vi "Dresser DXD Temp and Press Read Standalone.vi"(0 "Serial Port (COM1)":refnum<visa-resource-name>="COM1", 1 "Serial Baud Rate (19200)":u16(ring)=4 items=["1200", "2400", "4800", "9600", "19200", "38400", "57600", "115200"], 5 "DXD Address (1)":T2=1 min=1 max=99 step=1, 7 "Pressure Units (PSI)":T1(ring), 11 "Error In (no error)":errorcluster) -> (6 "Current Pressure":dbl min=-999999.0 max=999999.0 step=1e-05 format="%.2f", 8 "Current Temperature":dbl caption="°C" min=-999999.0 max=999999.0 step=1e-05 format="%.3f", 10 "Pressure Type":string, 15 "Error Out":errorcluster)   [LabVIEW 2015]
doc: "This getting started VI demonstrates how to continuously retrieve a pressure reading, with the selected units, and a temperature reading from the Dresser DXD Series pressure transducer at the specified address.\n\nSelect the serial port, serial baud rate, and DXD address prior to clicking the run arrow. \nThe pressure units selection can be changed while running.\nWritten by:\nBLOOMY CONTROLS, INC\nWINDSOR, CT 06095, USA\n860-298-9925\nwww.bloomy.com\nV2.0.0\nMay, 2002"
uses:
  Type Defs/DXD Address.ctl
panel:
  out "Heise Label (S/N)":string="000000"
  in  "Termination Character (T, <lf>)":bool=TRUE caption="<lf>\n<cr>"
  in  "Serial Stop Bits (1)":u16(ring)=10 items=["1.0"=10, "1.5"=15, "2.0"=20]
  in  "Serial Parity (even)":u16(ring)=2 items=["None", "Odd", "Even", "Mark", "Space"]
  in  "Serial Flow Control (None)":u16(ring) items=["None"=0, "XON/XOFF"=1, "RTS/CTS"=2, "DTR/DSR"=4]
  in  "Serial Data Bits (7)":u16=7
  out "Pressure Units":T1(ring)
  # "For instructions on the use of this VI, press Ctrl+H to display the help window and move the mouse over the icon, controls, and indicators"
  # "<---the unit selection can be changed while running"
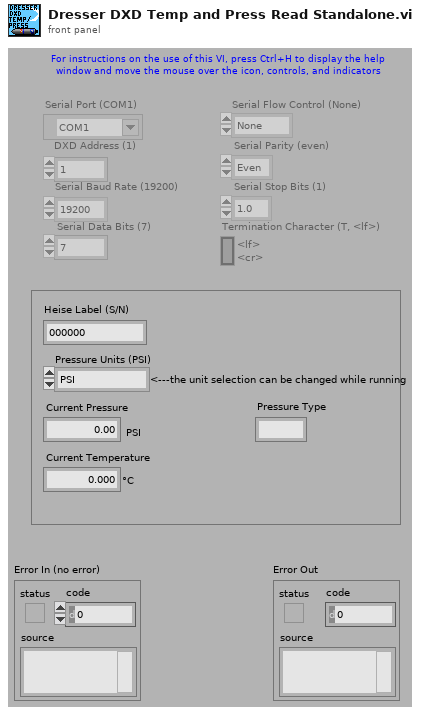
[diagram p1: front panel]
types:
  T1 = enum16{"PSI", "Bar", "cm H2O", "ft H2O", "hectoPascal", "in Hg", "in H2O", "kiloPascal", "milliBar", "mmHg", "MegaPascal", "Numeric Pressure"}
  T2 = typedef "DXD Address.ctl" = i32
  T3 = enum16{"Error status character set in bit 1 is returned", "No error status character (legacy mode)"}
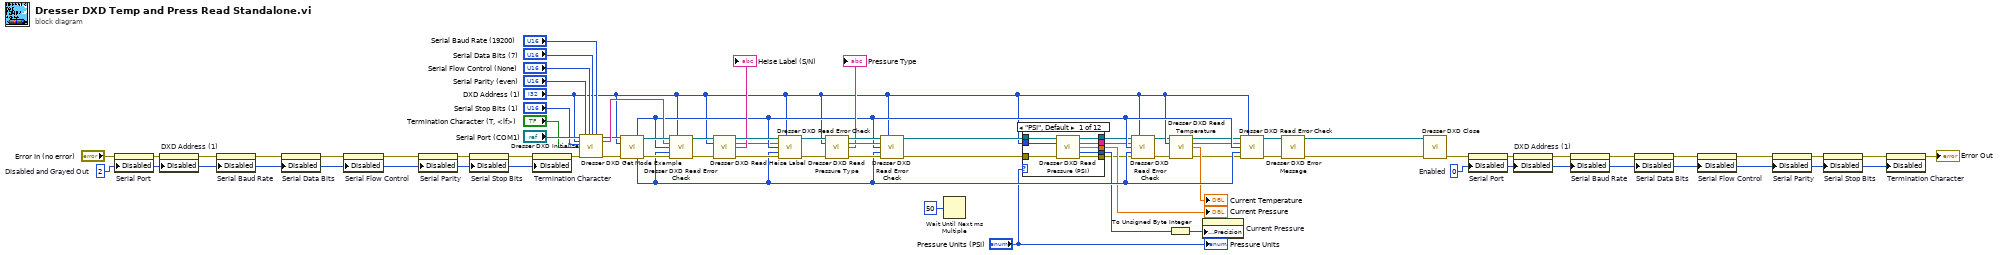
[diagram p0: block diagram]
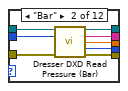
[diagram p2: hidden frame]
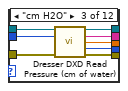
[diagram p3: hidden frame]
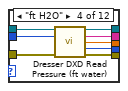
[diagram p4: hidden frame]
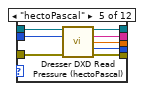
[diagram p5: hidden frame]
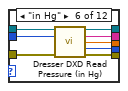
[diagram p6: hidden frame]
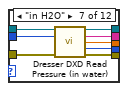
[diagram p7: hidden frame]
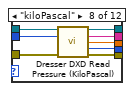
[diagram p8: hidden frame]
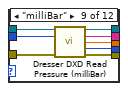
[diagram p9: hidden frame]
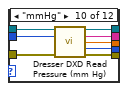
[diagram p10: hidden frame]
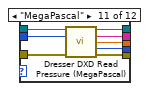
[diagram p11: hidden frame]
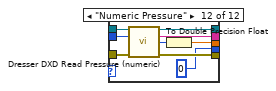
[diagram p12: hidden frame]
diagram:
  w39 = u8 0  # Enabled
  w45 = u8 2  # Disabled and Grayed Out
  n1 = property on="Serial Port" class="VISAName"(error in="Error In (no error)", "Disabled"=w45) -> (error out=w48:errorcluster)  [unwired: 1 in, 1 out]
  n2 = property on="DXD Address (1)" class="DigNum (strict)"(error in=w48, "Disabled"=w45) -> (error out=w47:errorcluster)  [unwired: 1 in, 1 out]
  n3 = property on="Serial Baud Rate" class="Ring (strict)"(error in=w47, "Disabled"=w45) -> (error out=w46:errorcluster)  [unwired: 1 in, 1 out]
  n4 = property on="Serial Data Bits" class="DigNum (strict)"(error in=w46, "Disabled"=w45) -> (error out=w44:errorcluster)  [unwired: 1 in, 1 out]
  n5 = property on="Serial Flow Control" class="Ring (strict)"(error in=w44, "Disabled"=w45) -> (error out=w43:errorcluster)  [unwired: 1 in, 1 out]
  n6 = property on="Serial Parity" class="Ring (strict)"(error in=w43, "Disabled"=w45) -> (error out=w42:errorcluster)  [unwired: 1 in, 1 out]
  n7 = property on="Serial Stop Bits" class="Ring (strict)"(error in=w42, "Disabled"=w45) -> (error out=w41:errorcluster)  [unwired: 1 in, 1 out]
  n8 = property on="Termination Character" class="Bool (strict)"(error in=w41, "Disabled"=w45) -> (error out=w40:errorcluster)  [unwired: 1 in, 1 out]
  n9 = call "Dresser DXD Initialize.vi"("Serial Port (COM1)"="Serial Port (COM1)", "DXD Address (1)"="DXD Address (1)", "Serial Stop Bits (1)"="Serial Stop Bits (1)", "Termination Character (T, <lf>)"="Termination Character (T, <lf>)", "error in (no error)"=w40, "Serial Parity (even)"="Serial Parity (even)", "Serial Flow Control (None)"="Serial Flow Control (None)", "Serial Data Bits (7)"="Serial Data Bits (7)", "Serial Baud Rate (19200)"="Serial Baud Rate (19200)") -> ("VISA session"=w28:refnum<visa-resource-name>, "Returned String"=w61:string, "Error Out"=w29:errorcluster)  [unwired: 8 in]
  n10 = call "Dresser DXD Get Mode Example.vi"("VISA session"=w28, "DXD Address (1)"="DXD Address (1)", "Error In (no error)"=w29) -> ("Bit 1 - Error Status Character"=w19:enum16{"ACK/NAK", "A/N"}, "dup VISA session"=w63:refnum<visa-resource-name>, "Bit 5 - Error Status Character"=w20:T3, "Error Out"=w62:errorcluster)  [unwired: 2 in, 7 out]
  n11 = call "Dresser DXD Read Error Check.vi"("VISA session"=w63, "DXD Address (1)"="DXD Address (1)", "Returned String (\"\")"=w61, "Mode Bit 1 - Error Status Character"=w19, "Mode Bit 5 - Error Status Character"=w20, "Error In (no error)"=w62) -> ("dup VISA session"=w27:refnum<visa-resource-name>, "Error Out"=w26:errorcluster)  [unwired: 6 in, 2 out]
  n12 = call "Dresser DXD Read Heise Label.vi"("VISA session"=w27, "DXD Address (1)"="DXD Address (1)", "Error In (no error)"=w26) -> ("dup VISA session"=w25:refnum<visa-resource-name>, "Returned String"=w18:string, "Heise Label (S/N)"=→"Heise Label (S/N)":string, "Error Out"=w24:errorcluster)  [unwired: 9 in]
  n13 = call "Dresser DXD Read Error Check.vi"("VISA session"=w25, "DXD Address (1)"="DXD Address (1)", "Returned String (\"\")"=w18, "Mode Bit 1 - Error Status Character"=w19, "Mode Bit 5 - Error Status Character"=w20, "Error In (no error)"=w24) -> ("dup VISA session"=w23:refnum<visa-resource-name>, "Error Out"=w22:errorcluster)  [unwired: 6 in, 2 out]
  n14 = call "Dresser DXD Read Pressure Type.vi"("VISA session"=w23, "DXD Address (1)"="DXD Address (1)", "Error In (no error)"=w22) -> ("dup VISA session"=w58:refnum<visa-resource-name>, "Returned String"=w56:string, "Pressure Type"=→"Pressure Type":string, "Error Out"=w60:errorcluster)  [unwired: 9 in]
  n15 = call "Dresser DXD Read Error Check.vi"("VISA session"=w58, "DXD Address (1)"="DXD Address (1)", "Returned String (\"\")"=w56, "Mode Bit 1 - Error Status Character"=w19, "Mode Bit 5 - Error Status Character"=w20, "Error In (no error)"=w60) -> ("dup VISA session"=w57:refnum<visa-resource-name>, "Error Out"=w59:errorcluster)  [unwired: 6 in, 2 out]
  n16 = Wait Until Next ms Multiple(millisecond multiple=u32 50) -> ()  [unwired: 1 out]
  n17 = case shown="\"PSI\", Default" "Pressure Units (PSI)" {
    tunnel: [w75 w78 w86 w94 w102 w110 w118 w126 w134 w142 w150 w160] -> w5
    tunnel: [w74 w81 w89 w97 w105 w113 w121 w129 w137 w145 w153 w162] -> w4
    tunnel: w57 -> [w73 w83 w91 w99 w107 w115 w123 w131 w139 w147 w155 w164]
    tunnel: w59 -> [w72 w82 w90 w98 w106 w114 w122 w130 w138 w146 w154 w163]
    tunnel: "DXD Address (1)" -> [w71 w77 w85 w93 w101 w109 w117 w125 w133 w141 w149 w159]
    tunnel: [w70 w80 w88 w96 w104 w112 w120 w128 w136 w144 w152 0 ("Pressure Decimal Position")] -> w14
    tunnel: [w69 w79 w87 w95 w103 w111 w119 w127 w135 w143 w151 w156] -> w13
    tunnel: [w68 w76 w84 w92 w100 w108 w116 w124 w132 w140 w148 w157] -> w1
    frame "PSI", Default {
      n18 = call "Dresser DXD Read Pressure (PSI).vi"("VISA session"=w73, "DXD Address (1)"=w71, "Error In (no error)"=w72) -> ("dup VISA session"=w75:refnum<visa-resource-name>, "Returned String"=w68:string, "Current Pressure (PSI)"=w69:dbl, "Pressure Decimal Position"=w70:i32, "Error Out"=w74:errorcluster)  [unwired: 8 in]
    }
    frame "Bar" {
      n19 = call "Dresser DXD Read Pressure (Bar).vi"("VISA session"=w83, "DXD Address (1)"=w77, "Error In (no error)"=w82) -> ("dup VISA session"=w78:refnum<visa-resource-name>, "Returned String"=w76:string, "Current Pressure (Bar)"=w79:dbl, "Pressure Decimal Position"=w80:i32, "Error Out"=w81:errorcluster)  [unwired: 8 in]
    }
    frame "cm H2O" {
      n20 = call "Dresser DXD Read Pressure (cm of water).vi"("VISA session"=w91, "DXD Address (1)"=w85, "Error In (no error)"=w90) -> ("dup VISA session"=w86:refnum<visa-resource-name>, "Returned String"=w84:string, "Current Pressure (cm of water)"=w87:dbl, "Pressure Decimal Position"=w88:i32, "Error Out"=w89:errorcluster)  [unwired: 8 in]
    }
    frame "ft H2O" {
      n21 = call "Dresser DXD Read Pressure (ft water).vi"("VISA session"=w99, "DXD Address (1)"=w93, "Error In (no error)"=w98) -> ("dup VISA session"=w94:refnum<visa-resource-name>, "Returned String"=w92:string, "Current Pressure (ft water)"=w95:dbl, "Pressure Decimal Position"=w96:i32, "Error Out"=w97:errorcluster)  [unwired: 8 in]
    }
    frame "hectoPascal" {
      n22 = call "Dresser DXD Read Pressure (hectoPascal).vi"("VISA session"=w107, "DXD Address (1)"=w101, "Error In (no error)"=w106) -> ("dup VISA session"=w102:refnum<visa-resource-name>, "Returned String"=w100:string, "Current Pressure (hectoPascal)"=w103:dbl, "Pressure Decimal Position"=w104:i32, "Error Out"=w105:errorcluster)  [unwired: 8 in]
    }
    frame "in Hg" {
      n23 = call "Dresser DXD Read Pressure (in Hg).vi"("VISA session"=w115, "DXD Address (1)"=w109, "Error In (no error)"=w114) -> ("dup VISA session"=w110:refnum<visa-resource-name>, "Returned String"=w108:string, "Current Pressure (in Hg)"=w111:dbl, "Pressure Decimal Position"=w112:i32, "Error Out"=w113:errorcluster)  [unwired: 8 in]
    }
    frame "in H2O" {
      n24 = call "Dresser DXD Read Pressure (in water).vi"("VISA session"=w123, "DXD Address (1)"=w117, "Error In (no error)"=w122) -> ("dup VISA session"=w118:refnum<visa-resource-name>, "Returned String"=w116:string, "Current Pressure (in H2O)"=w119:dbl, "Pressure Decimal Position"=w120:i32, "Error Out"=w121:errorcluster)  [unwired: 8 in]
    }
    frame "kiloPascal" {
      n25 = call "Dresser DXD Read Pressure (KiloPascal).vi"("VISA session"=w131, "DXD Address (1)"=w125, "Error In (no error)"=w130) -> ("dup VISA session"=w126:refnum<visa-resource-name>, "Returned String"=w124:string, "Current Pressure (KiloPascal)"=w127:dbl, "Pressure Decimal Position"=w128:i32, "Error Out"=w129:errorcluster)  [unwired: 8 in]
    }
    frame "milliBar" {
      n26 = call "Dresser DXD Read Pressure (milliBar).vi"("VISA session"=w139, "DXD Address (1)"=w133, "Error In (no error)"=w138) -> ("dup VISA session"=w134:refnum<visa-resource-name>, "Returned String"=w132:string, "Current Pressure (milliBar)"=w135:dbl, "Pressure Decimal Position"=w136:i32, "Error Out"=w137:errorcluster)  [unwired: 8 in]
    }
    frame "mmHg" {
      n27 = call "Dresser DXD Read Pressure (mm Hg).vi"("VISA session"=w147, "DXD Address (1)"=w141, "Error In (no error)"=w146) -> ("dup VISA session"=w142:refnum<visa-resource-name>, "Returned String"=w140:string, "Current Pressure (mm Hg)"=w143:dbl, "Pressure Decimal Position"=w144:i32, "Error Out"=w145:errorcluster)  [unwired: 8 in]
    }
    frame "MegaPascal" {
      n28 = call "Dresser DXD Read Pressure (MegaPascal).vi"("VISA session"=w155, "DXD Address (1)"=w149, "Error In (no error)"=w154) -> ("dup VISA session"=w150:refnum<visa-resource-name>, "Returned String"=w148:string, "Current Pressure (MegaPascal)"=w151:dbl, "Pressure Decimal Position"=w152:i32, "Error Out"=w153:errorcluster)  [unwired: 8 in]
    }
    frame "Numeric Pressure" {
      n29 = call "Dresser DXD Read Pressure (numeric).vi"("VISA session"=w164, "DXD Address (1)"=w159, "Error In (no error)"=w163) -> ("dup VISA session"=w160:refnum<visa-resource-name>, "Returned String"=w157:string, "Current Numeric Value"=w161:i32, "Error Out"=w162:errorcluster)  [unwired: 9 in]
      n30 = To Double Precision Float(number=w161) -> (double precision float=w156:dbl)
    }
  }
  "Current Pressure" <- w13
  n31 = call "Dresser DXD Read Error Check.vi"("VISA session"=w5, "DXD Address (1)"="DXD Address (1)", "Returned String (\"\")"=w1, "Mode Bit 1 - Error Status Character"=w19, "Mode Bit 5 - Error Status Character"=w20, "Error In (no error)"=w4) -> ("dup VISA session"=w2:refnum<visa-resource-name>, "Error Out"=w3:errorcluster)  [unwired: 6 in, 2 out]
  n32 = To Unsigned Byte Integer(number=w14) -> (unsigned 8bit integer=w16:u8)
  n33 = call "Dresser DXD Read Temperature.vi"("VISA session"=w2, "DXD Address (1)"="DXD Address (1)", "Error In (no error)"=w3) -> ("dup VISA session"=w10:refnum<visa-resource-name>, "Returned String"=w6:string, "Current Temperature (°C)"=→"Current Temperature":dbl, "Error Out"=w9:errorcluster)  [unwired: 9 in]
  n34 = property on="Current Pressure" class="DigNum (strict)"("Display Format:Precision"=w16) -> ()  [unwired: 2 in, 2 out]
  n35 = call "Dresser DXD Read Error Check.vi"("VISA session"=w10, "DXD Address (1)"="DXD Address (1)", "Returned String (\"\")"=w6, "Mode Bit 1 - Error Status Character"=w19, "Mode Bit 5 - Error Status Character"=w20, "Error In (no error)"=w9) -> ("dup VISA session"=w8:refnum<visa-resource-name>, "Error Out"=w7:errorcluster)  [unwired: 6 in, 2 out]
  n36 = call "Dresser DXD Error Message.vi"("VISA session"=w8, "Error In (no error)"=w7) -> ("dup VISA session"=w67:refnum<visa-resource-name>, "Error Out"=w66:errorcluster)  [unwired: 9 in, 3 out]
  n37 = call "Dresser DXD Close.vi"("VISA session"=w67, "Error In (no error)"=w66) -> ("Error Out"=w38:errorcluster)  [unwired: 13 in]
  n38 = property on="Serial Port" class="VISAName"(error in=w38, "Disabled"=w39) -> (error out=w36:errorcluster)  [unwired: 1 in, 1 out]
  n39 = property on="DXD Address (1)" class="DigNum (strict)"(error in=w36, "Disabled"=w39) -> (error out=w35:errorcluster)  [unwired: 1 in, 1 out]
  n40 = property on="Serial Baud Rate" class="Ring (strict)"(error in=w35, "Disabled"=w39) -> (error out=w34:errorcluster)  [unwired: 1 in, 1 out]
  n41 = property on="Serial Data Bits" class="DigNum (strict)"(error in=w34, "Disabled"=w39) -> (error out=w33:errorcluster)  [unwired: 1 in, 1 out]
  n42 = property on="Serial Flow Control" class="Ring (strict)"(error in=w33, "Disabled"=w39) -> (error out=w32:errorcluster)  [unwired: 1 in, 1 out]
  n43 = property on="Serial Parity" class="Ring (strict)"(error in=w32, "Disabled"=w39) -> (error out=w31:errorcluster)  [unwired: 1 in, 1 out]
  n44 = property on="Serial Stop Bits" class="Ring (strict)"(error in=w31, "Disabled"=w39) -> (error out=w30:errorcluster)  [unwired: 1 in, 1 out]
  n45 = property on="Termination Character" class="Bool (strict)"(error in=w30, "Disabled"=w39) -> (error out=→"Error Out":errorcluster)  [unwired: 1 in, 1 out]
  "Pressure Units" <- "Pressure Units (PSI)"
